vi "Settings Dialog.vi"(8 "error in (no error)":errorcluster, 11 "Settings in":T1 {"Hardware Configuration"."Sample mode" items=["Continuous Samples"=10123]}) -> (0 "error out":errorcluster, 1 "Cancelled?":bool, 2 "UI Refresh Needed?":bool, 3 "Settings out":T1 {"Hardware Configuration"."Sample mode" items=["Continuous Samples"=10123]})   [LabVIEW 2018, in "Settings.lvlib"]
doc: "Dialog for selecting user specified settings."
uses:
  Settings.lvlib
  Settings.ctl
  Acquisition/Hardware Configuration.ctl
  Logging/Logging Configuration.ctl
  <vilib>/Utility/xml.llb/Write to XML File(string).vi
  Acquisition/Acquisition.lvlib
  Logging/Logging.lvlib
panel:
  in  "Counter Channel":tag="SimDev1/ai0"
  in  "Counter Name":string="Battery Voltage"
  in  "Scale Channel 3":dbl
  in  "Scale Channel 2":dbl
  in  "Scale Channel 1":dbl
  in  "Offset Channel 3":dbl
  in  "Offset Channel 2":dbl
  in  "Offset Channel 1":dbl
  in  "Sample Mode":u16(ring)=10123 items=["Finite Samples"=10178, "Continuous Samples"=10123, "Hardware Timed Single Point"=12522]
  in  "Samples per channel":u32
  in  "Samples per second":dbl=1000.0
  in  "Sample time in ms":u32=10
  in  "Channel 3 Name":string="Brake torque"
  in  "Channel 2 Name":string="Battery Current"
  in  "Channel 1 Name":string="Battery Voltage"
  in  "Channel 3":tag="SimDev1/ai2"
  in  "Channel 2":tag="SimDev1/ai1"
  in  "Log File Path":path
  in  "Channel 1":tag="SimDev1/ai0"
  in  "Cancel Button":bool
  in  "OK Button":bool
  # "Non visible portion of dialog (needed for connector pane)."
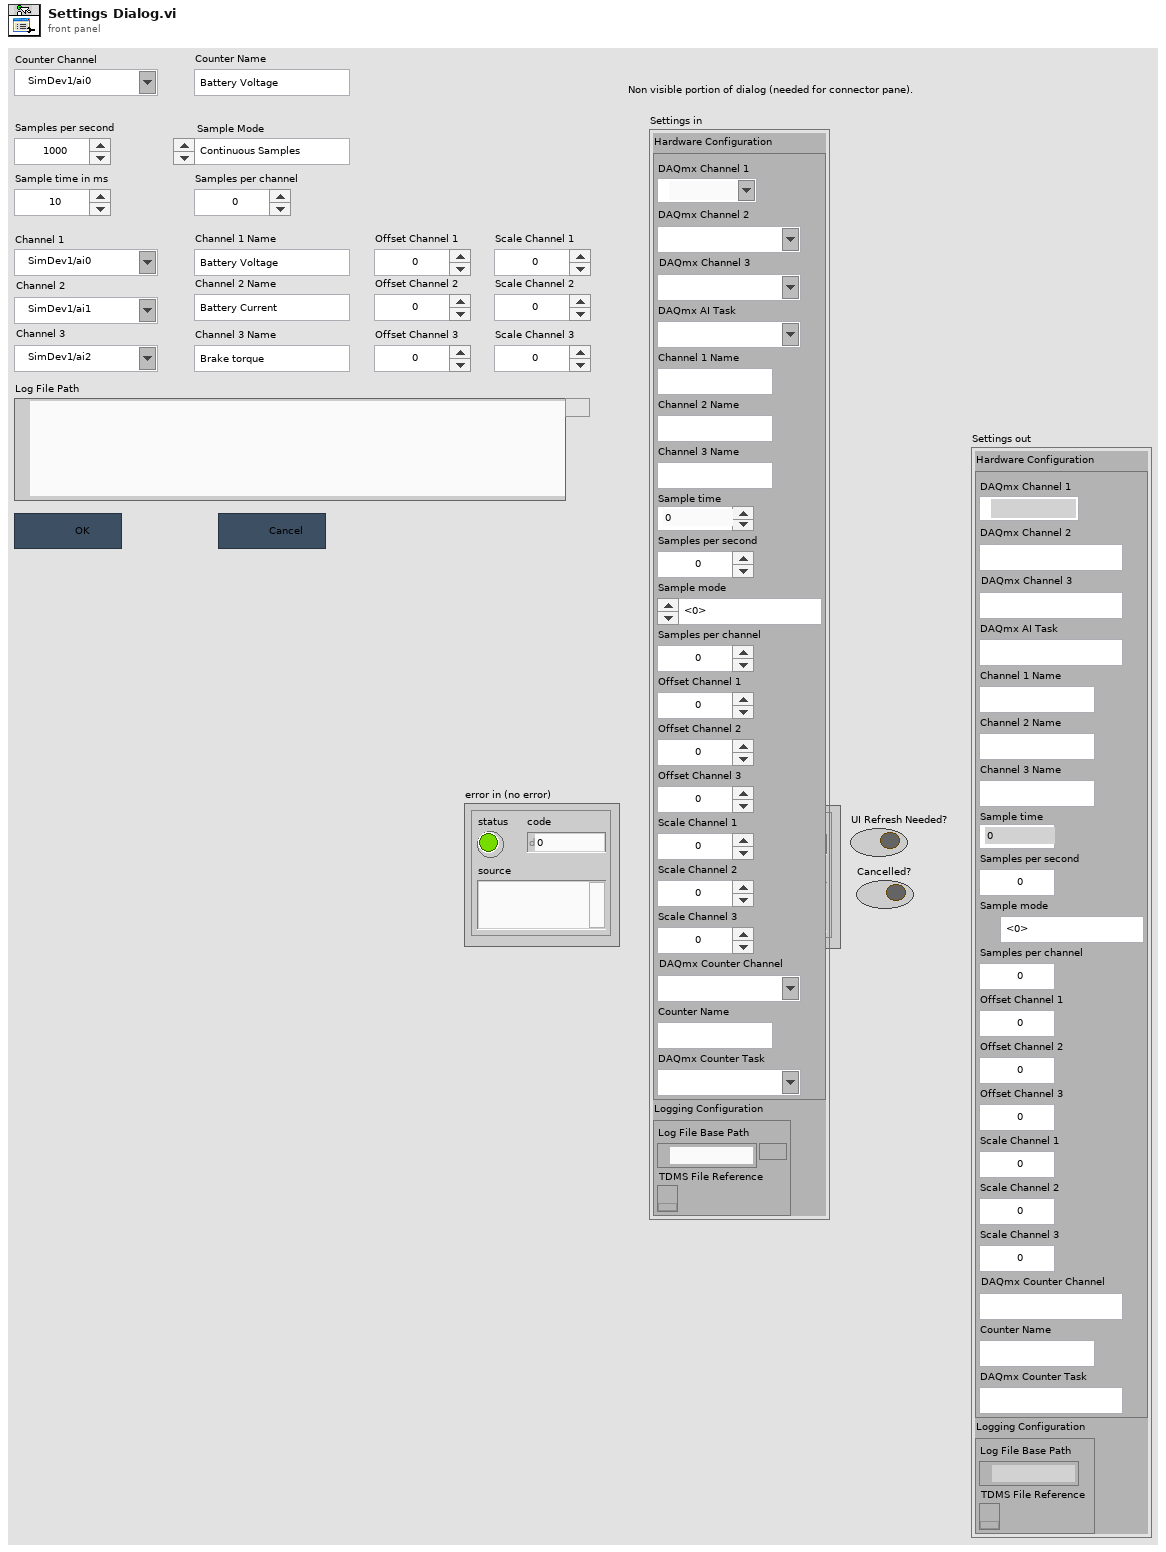
[diagram p1: front panel]
types:
  T1 = typedef "Settings.lvlib/Settings.ctl" = cluster{"Hardware Configuration":T2, "Logging Configuration":T3}
  T2 = typedef "Acquisition.lvlib/Hardware Configuration.ctl" = cluster{"DAQmx Channel 1":tag, "DAQmx Channel 2":tag, "DAQmx Channel 3":tag, "DAQmx AI Task":refnum<k21>, "Channel 1 Name":string, "Channel 2 Name":string, "Channel 3 Name":string, "Sample time":u32, "Samples per second":dbl, "Sample mode":u16, "Samples per channel":i32, "Offset Channel 1":dbl, "Offset Channel 2":dbl, "Offset Channel 3":dbl, "Scale Channel 1":dbl, "Scale Channel 2":dbl, "Scale Channel 3":dbl, "DAQmx Counter Channel":tag, "Counter Name":string, "DAQmx Counter Task":refnum<k21>}
  T3 = typedef "Logging.lvlib/Logging Configuration.ctl" = cluster{"Log File Base Path":path, "TDMS File Reference":refnum<k34>}
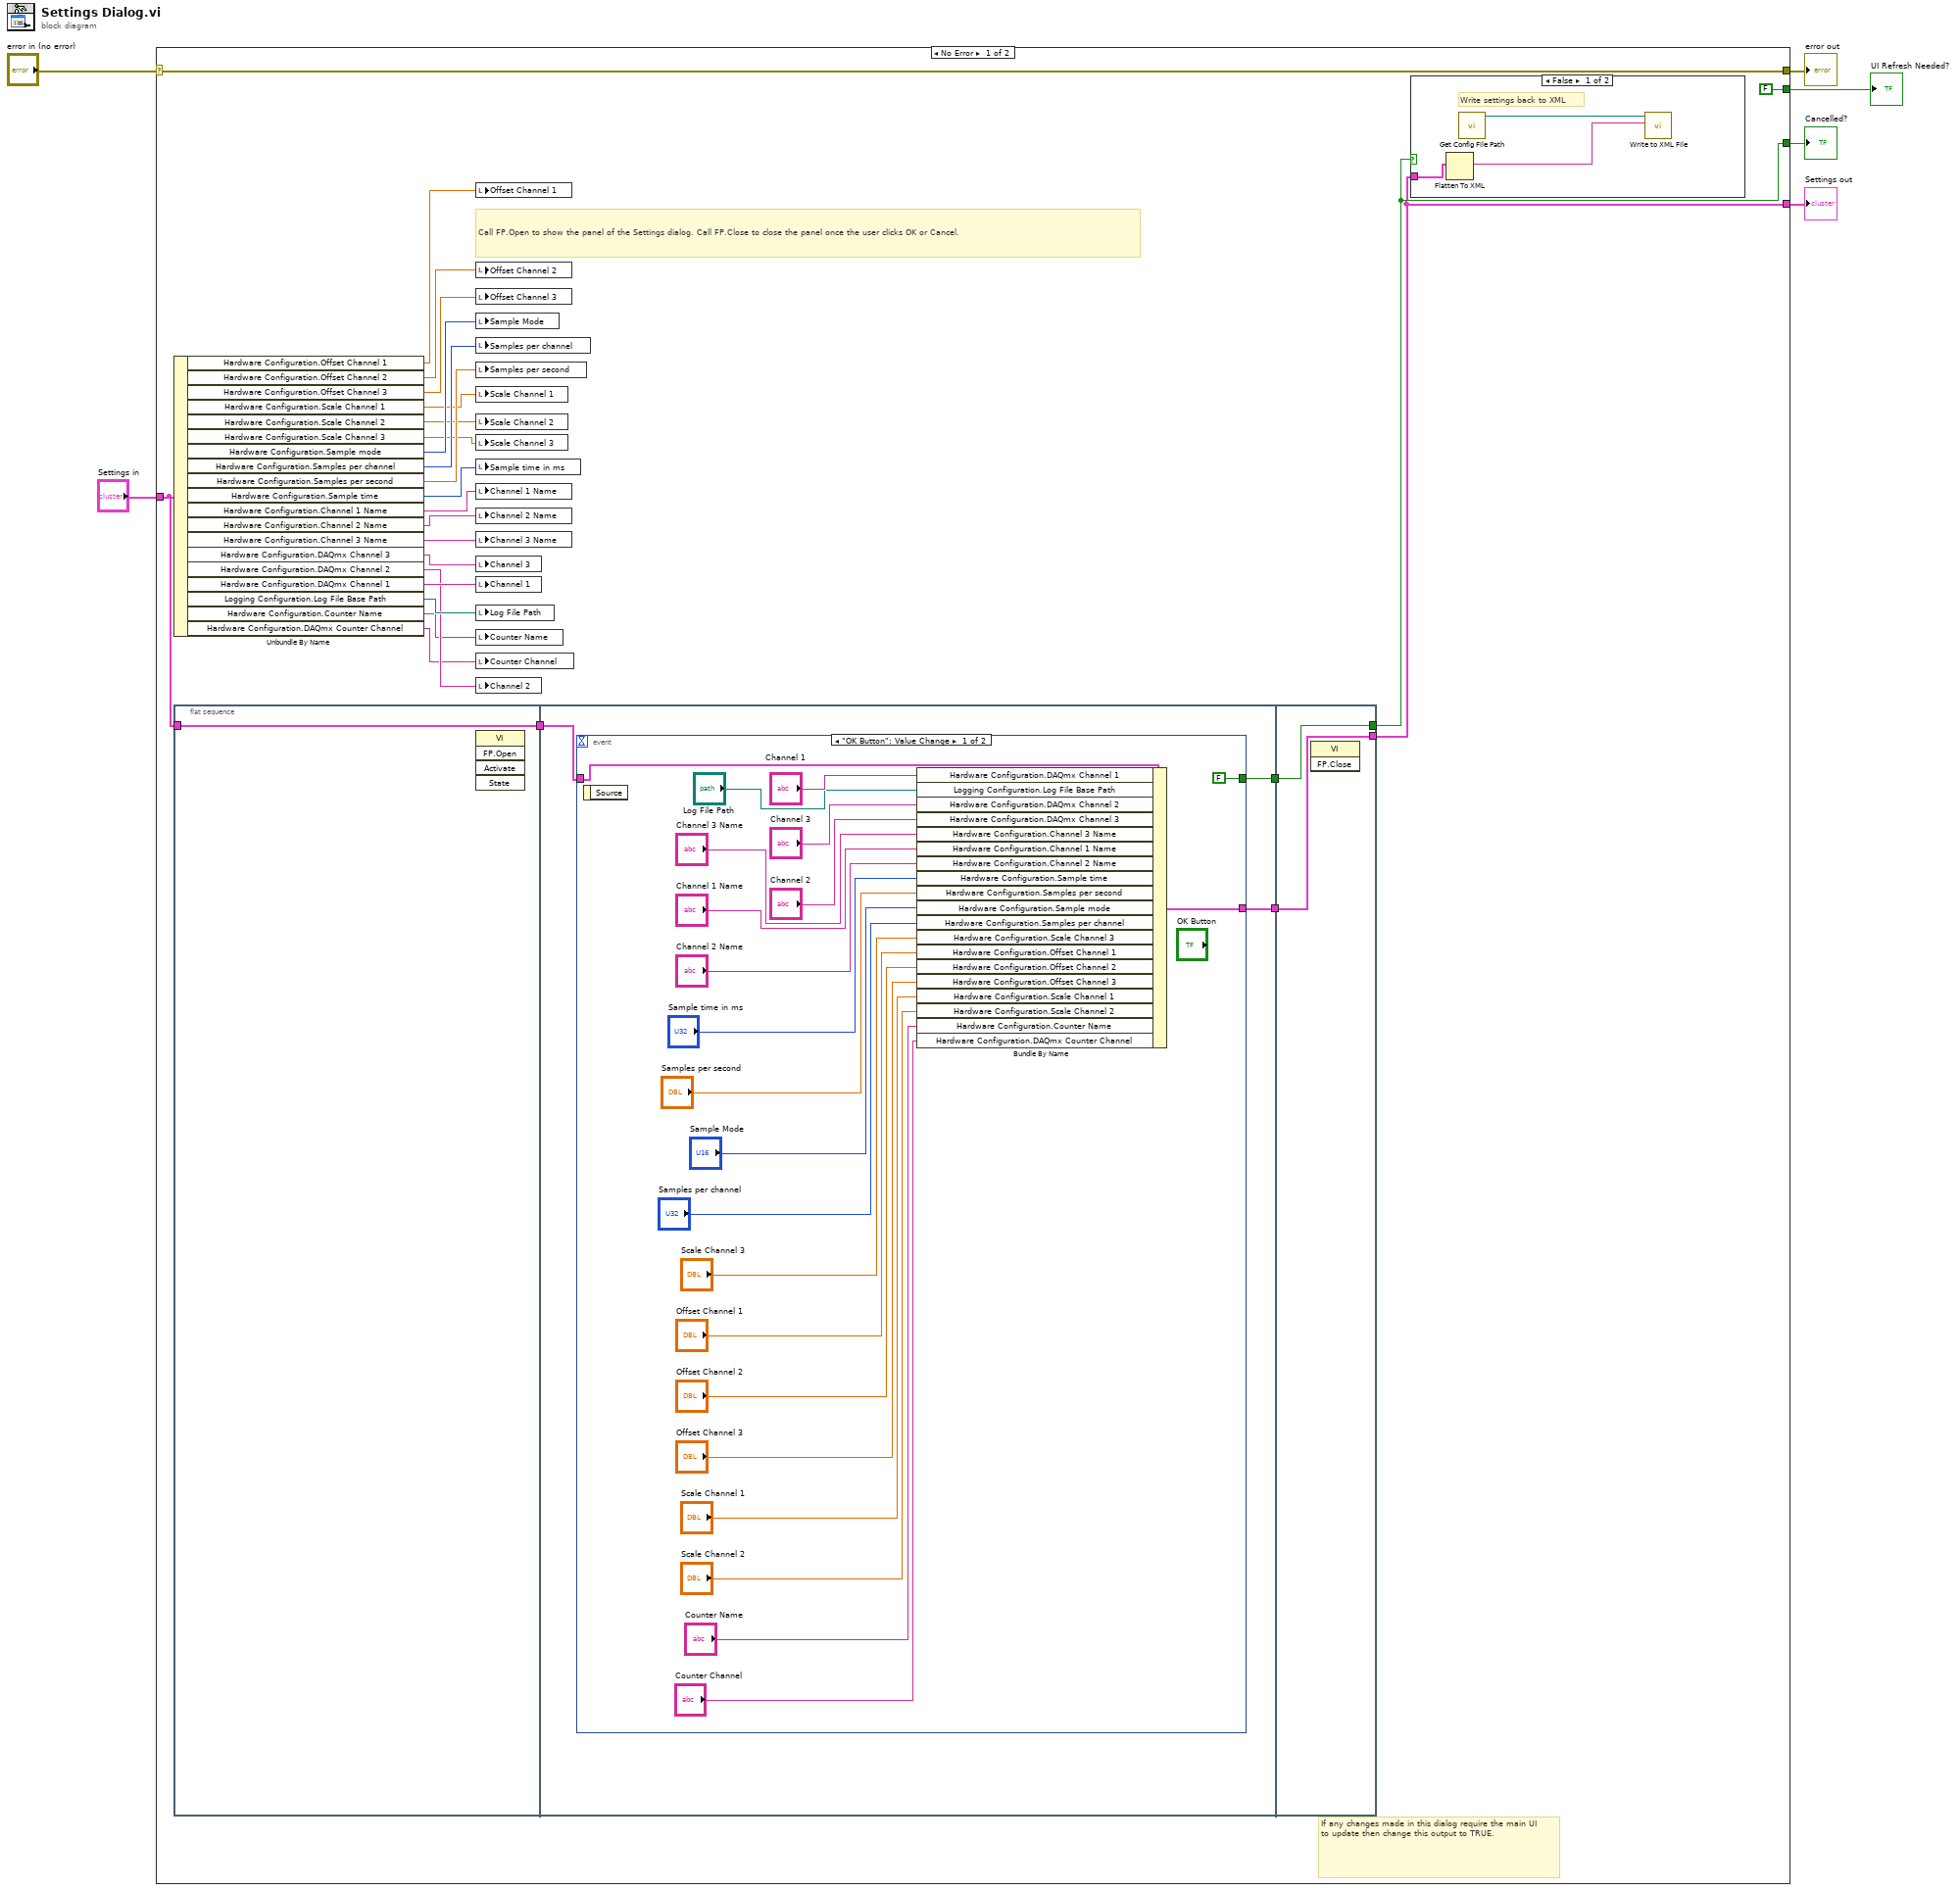
[diagram p0: block diagram]
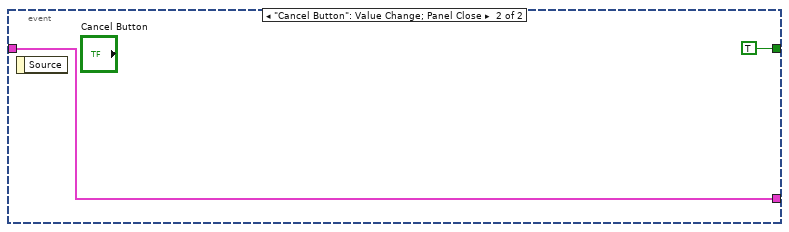
[diagram p2: hidden frame]
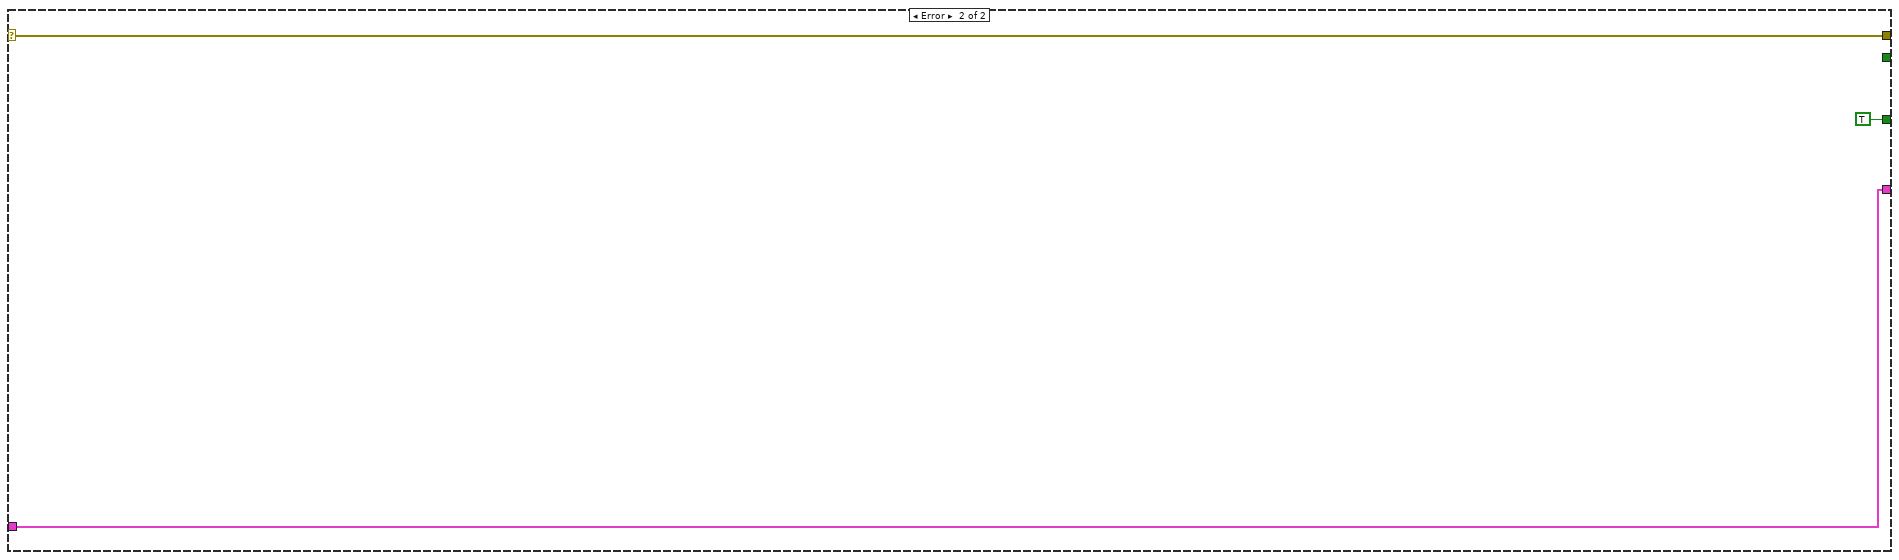
[diagram p4: hidden frame]
diagram:
  n1 = case shown="No Error" "error in (no error)" {
    selector: "error in (no error)" -> [w33 w69]
    tunnel: [w33 w69] -> w5
    tunnel: "Settings in" -> [w29 w68]
    tunnel: [w30 w68] -> w3
    tunnel: [FALSE ("UI Refresh Needed?") _] -> w2
    tunnel: [w31 TRUE ("UI Refresh Needed?")] -> w1
    frame No Error {
      # "Call FP.Open to show the panel of the Settings dialog. Call FP.Close to close the panel once the user clicks OK or Cancel."
      # "If any changes made in this dialog require the main UI to update then change this output to TRUE."
      n2 = Unbundle By Name(w29) -> ("Hardware Configuration.Offset Channel 1"=w13:dbl, "Hardware Configuration.Offset Channel 2"=w11:dbl, "Hardware Configuration.Offset Channel 3"=w14:dbl, "Hardware Configuration.Scale Channel 1"=w9:dbl, "Hardware Configuration.Scale Channel 2"=w10:dbl, "Hardware Configuration.Scale Channel 3"=w12:dbl, "Hardware Configuration.Sample mode"=w15:u16, "Hardware Configuration.Samples per channel"=w16:i32, "Hardware Configuration.Samples per second"=w17:dbl, "Hardware Configuration.Sample time"=w18:u32, "Hardware Configuration.Channel 1 Name"=w19:string, "Hardware Configuration.Channel 2 Name"=w20:string, "Hardware Configuration.Channel 3 Name"=w21:string, "Hardware Configuration.DAQmx Channel 3"=w22:tag, "Hardware Configuration.DAQmx Channel 2"=w23:tag, "Hardware Configuration.DAQmx Channel 1"=w28:tag, "Logging Configuration.Log File Base Path"=w27:path, "Hardware Configuration.Counter Name"=w7:string, "Hardware Configuration.DAQmx Counter Channel"=w8:tag)
      n3 = flat-sequence {
        tunnel: w29 -> [w34]
        tunnel: [w34] -> w26
        tunnel: w26 -> [w35]
        tunnel: [w37] -> w25
        tunnel: [w36] -> w24
        tunnel: [w62] -> w30
        tunnel: [w63] -> w31
        tunnel: w25 -> [w63]
        tunnel: w24 -> [w62]
        frame #0 {
          n4 = invoke class="VI" method="FP.Open"() -> ()  [unwired: 5 in, 5 out]
        }
        frame #1 {
          n5 = event shown="[0] \"OK Button\": Value Change" {
            selector: _ -> [_ _]
            dyn-events: _ -> [_ _]
            timeout: _ -> [_ _]
            tunnel: [w57 w61] -> w36
            tunnel: w35 -> [w58 w61]
            tunnel: [FALSE ("UI Refresh Needed?") TRUE ("UI Refresh Needed?")] -> w37
            event "OK Button": Value Change {
              n6 = event-data() -> ()  [unwired: 1 in, 1 out]
              n7 = Bundle By Name(cluster=w58, "Hardware Configuration.DAQmx Channel 1"="Channel 1", "Logging Configuration.Log File Base Path"="Log File Path", "Hardware Configuration.DAQmx Channel 2"="Channel 3", "Hardware Configuration.DAQmx Channel 3"="Channel 2", "Hardware Configuration.Channel 3 Name"="Channel 3 Name", "Hardware Configuration.Channel 1 Name"="Channel 1 Name", "Hardware Configuration.Channel 2 Name"="Channel 2 Name", "Hardware Configuration.Sample time"="Sample time in ms", "Hardware Configuration.Samples per second"="Samples per second", "Hardware Configuration.Sample mode"="Sample Mode", "Hardware Configuration.Samples per channel"="Samples per channel", "Hardware Configuration.Scale Channel 3"="Scale Channel 3", "Hardware Configuration.Offset Channel 1"="Offset Channel 1", "Hardware Configuration.Offset Channel 2"="Offset Channel 2", "Hardware Configuration.Offset Channel 3"="Offset Channel 3", "Hardware Configuration.Scale Channel 1"="Scale Channel 1", "Hardware Configuration.Scale Channel 2"="Scale Channel 2", "Hardware Configuration.Counter Name"="Counter Name", "Hardware Configuration.DAQmx Counter Channel"="Counter Channel") -> (w57:T1)
            }
            event "Cancel Button": Value Change; Panel Close {
              n8 = event-data() -> ()  [unwired: 1 in, 1 out]
            }
          }
        }
        frame #2 {
          n9 = invoke class="VI" method="FP.Close"() -> ()  [unwired: 3 in, 3 out]
        }
      }
      n10 = local write "Offset Channel 1"(w13) -> ()
      n11 = local write "Offset Channel 2"(w11) -> ()
      n12 = local write "Offset Channel 3"(w14) -> ()
      n13 = local write "Sample Mode"(w15) -> ()
      n14 = local write "Samples per channel"(w16) -> ()
      n15 = local write "Samples per second"(w17) -> ()
      n16 = local write "Scale Channel 1"(w9) -> ()
      n17 = local write "Scale Channel 2"(w10) -> ()
      n18 = local write "Scale Channel 3"(w12) -> ()
      n19 = local write "Sample time in ms"(w18) -> ()
      n20 = local write "Channel 1 Name"(w19) -> ()
      n21 = local write "Channel 2 Name"(w20) -> ()
      n22 = local write "Channel 3 Name"(w21) -> ()
      n23 = local write "Channel 3"(w22) -> ()
      n24 = local write "Channel 1"(w28) -> ()
      n25 = local write "Log File Path"(w27) -> ()
      n26 = local write "Counter Name"(w7) -> ()
      n27 = local write "Counter Channel"(w8) -> ()
      n28 = local write "Channel 2"(w23) -> ()
      n29 = case shown="False" w31 {
        tunnel: w30 -> [w65 _]
        frame False {
          # "Write settings back to XML"
          n30 = Flatten To XML(anything=w65) -> (xml string=w64:string)
          n31 = call "Get Config File Path.vi"() -> ("XML File Path"=w66:path)  [unwired: 10 in, 1 out]
          n32 = call-poly <vilib>:"Write to XML File.vi"("XML Input"=w64, "XML File Path"=w66) -> ()  [unwired: 7 in, 3 out]
        }
        frame True {
        }
      }
    }
    frame Error {
    }
  }
  "UI Refresh Needed?" <- w2
  "error out" <- w5
  "Settings out" <- w3
  "Cancelled?" <- w1
